vi "XBrio write.vi"() -> ()   [LabVIEW 2013]
uses:
  C:/Program Files (x86)/National Instruments/LabVIEW 2013/examples/Instrument IO/Serial/support/Serial - Settings.ctl
  <vilib>/Instr/_visa.llb/VISA Configure Serial Port (Instr).vi
panel:
  in  "bytes to read":dbl
  in  "String":string
  out "Input sting HEX":string
  in  "VISA resource name":refnum<visa-resource-name>="COM1"
  in  "delay before read (ms)":u32=500
  out "bytes read":u32
  in  "Serial Settings":T1={"baud rate"=9600, "data bits"=8, "parity"=enum."None", "stop bits"=10, "flow control"=0} {"flow control" items=["None"=0, "XON/XOFF"=1, "RTS/CTS"=2, "DTR/DSR"=4]; "stop bits" items=["1.0"=10, "1.5"=15, "2.0"=20]; "data bits" min=5 max=8 step=1; "baud rate" items=["75"=75, "110"=110, "134"=134, "150"=150, "300"=300, "600"=600, "1200"=1200, "1800"=1800, "2400"=2400, "4800"=4800, "7200"=7200, "9600"=9600, "14400"=14400, "19200"=19200, "28800"=28800, "38400"=38400, "56000"=56000, "57600"=57600, "115200"=115200, "128000"=128000, "230400"=230400]}
  in  "?":bool
  out "Response":string
  out "String to U16":u16[](array[numeric])
  out "IR2":u16
  out "IR1":u16
  out "Encoder1":u16
  out "Encoder2":u16
  # "Example to send dec 100 \nhttp://www.makershed.com/v/vspfiles/assets/images/122-32450-xbeetutorial-v1.0.1.pdf\n7E00 0901 0150 0100 3130 300D 0E"
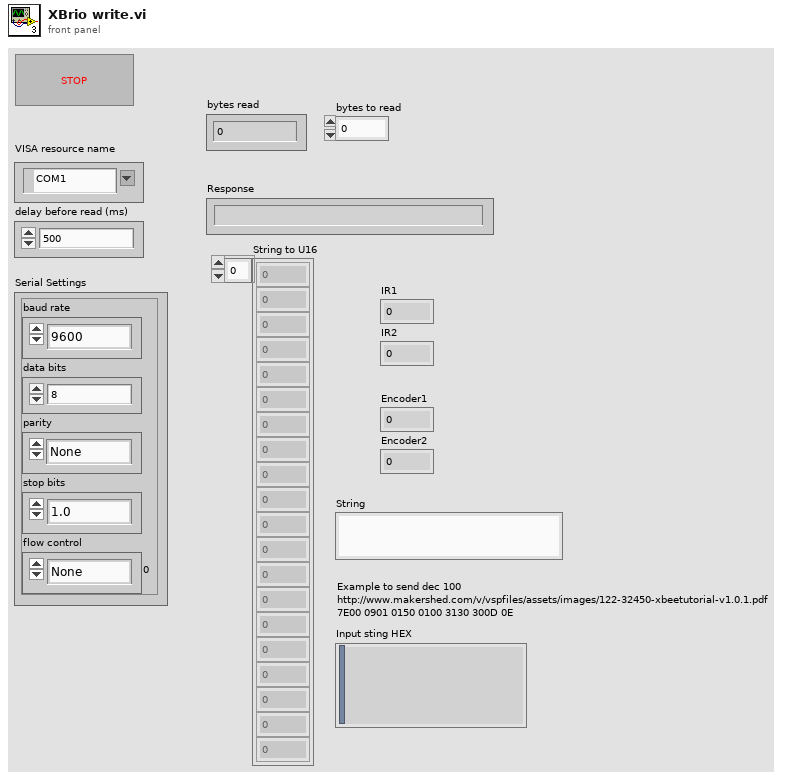
[diagram p1: front panel]
types:
  T1 = typedef "Serial - Settings.ctl" = cluster{"baud rate":u32, "data bits":u16, "parity":enum16{"None", "Odd", "Even", "Mark", "Space"}, "stop bits":u16, "flow control":u16}
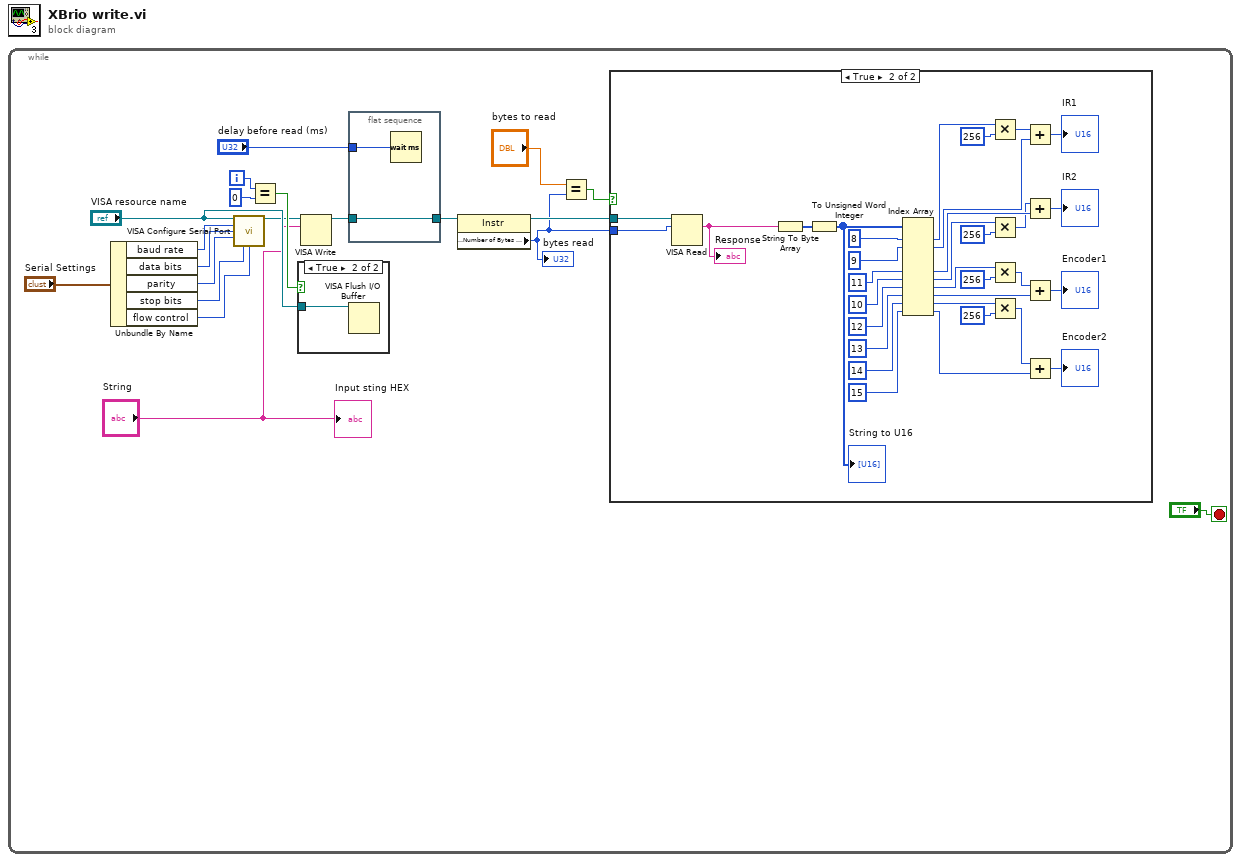
[diagram p0: block diagram]
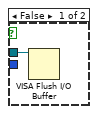
[diagram p2: hidden frame]
diagram:
  n1 = while {
    i -> [w11]
    stop <- "?" stop-if-true
    n2 = Unbundle By Name("Serial Settings") -> ("baud rate"=w18:u32, "data bits"=w17:u16, "parity"=w16:enum16{"None", "Odd", "Even", "Mark", "Space"}, "stop bits"=w15:u16, "flow control"=w14:u16)
    n3 = call-poly "VISA Configure Serial Port"("VISA resource name"="VISA resource name", "baud rate (9600)"=w18, "data bits (8)"=w17, "parity (0:none)"=w16, "stop bits (10: 1 bit)"=w15, "flow control (0:none)"=w14) -> ("VISA resource name out"=w6:refnum<visa-resource-name>)  [unwired: 3 in, 6 out]
    n4 = Equal?(x=w11, y=0) -> (x = y?=w9:bool)
    n5 = case shown="True" w9 {
      tunnel: "VISA resource name" -> [_ w55]
      frame False {
      }
      frame True {
        n6 = VISA Flush I/O Buffer(VISA resource name=w55) -> ()  [unwired: 2 in, 2 out]
      }
    }
    n7 = VISA Write(VISA resource name=w6, write buffer="String") -> (VISA resource name out=w5:refnum<visa-resource-name>)  [unwired: 1 in, 2 out]
    n8 = flat-sequence {
      tunnel: w5 -> [w56]
      tunnel: [w56] -> w13
      tunnel: "delay before read (ms)" -> [w57]
      frame #0 {
        n9 = Wait (ms)(milliseconds to wait=w57) -> ()  [unwired: 1 out]
      }
    }
    n10 = property class="Instr"(reference=w13) -> (reference out=w7:refnum<visa-resource-name>, "Serial Settings:Number of Bytes at Serial Port"=w1:u32)  [unwired: 1 in, 1 out]
    "bytes read" <- w1
    n11 = Equal?(x="bytes to read", y=w1) -> (x = y?=w3:bool)
    n12 = case shown="True" w3 {
      tunnel: w1 -> [_ w23]
      tunnel: w7 -> [w21 w22]
      frame False {
        n13 = VISA Flush I/O Buffer(VISA resource name=w21) -> ()  [unwired: 2 in, 2 out]
      }
      frame True {
        n14 = VISA Read(VISA resource name=w22, byte count=w23) -> (read buffer=w25:string)  [unwired: 1 in, 3 out]
        "Response" <- w25
        n15 = String To Byte Array(string=w25) -> (unsigned byte array=w26:u8[])
        n16 = To Unsigned Word Integer(number=w26) -> (unsigned 16bit integer=w24:u16[])
        "String to U16" <- w24
        n17 = Index Array(array=w24, index #1=8 ("index"), index #2=9 ("index"), index #5=11, index #6=10 ("index"), index #7=12 ("index"), index #8=13 ("index"), index #9=14 ("index"), index #10=15 ("index")) -> (element #1=w34:u16, element #2=w37:u16, element #5=w31:u16, element #6=w29:u16, element #7=w42:u16, element #8=w43:u16, element #9=w49:u16, element #10=w50:u16)  [unwired: 2 in, 2 out]
        n18 = Multiply(x=w34, y=u16 256) -> (x*y=w36:u16)
        n19 = Multiply(x=w29, y=u16 256) -> (x*y=w27:u16)
        n20 = Multiply(x=w42, y=u16 256) -> (x*y=w38:u16)
        n21 = Multiply(x=w49, y=u16 256) -> (x*y=w48:u16)
        n22 = Add(x=w36, y=w37) -> (x+y=→"IR1":u16)
        n23 = Add(x=w27, y=w31) -> (x+y=→"IR2":u16)
        n24 = Add(x=w38, y=w43) -> (x+y=→"Encoder1":u16)
        n25 = Add(x=w48, y=w50) -> (x+y=→"Encoder2":u16)
      }
    }
    "Input sting HEX" <- "String"
  }
